vi "Init Messaging.vi"(8 "error in (no error)":errorcluster, 11 "LV Server in":refnum<class "LV Server.lvclass">) -> (0 "error out":errorcluster, 3 "LV Server out":refnum<class "LV Server.lvclass">)   [LabVIEW 2020, in "LV Server.lvclass"]
uses:
  LV Server.lvclass
  <vilib>/IlluminatedG/IG WebSocket Stream/Stream-Websocket/Websocket Server/Websocket Server.lvclass
  C:/Program Files (x86)/National Instruments/LabVIEW 2020/vi.lib/IlluminatedG/lv-stream/Endpoint/Endpoint.lvclass
  <vilib>/IlluminatedG/lv-stream-tcp/TCP Server/TCP Server.lvclass
  Common/Message ID.ctl
  <vilib>/IlluminatedG/lv-msg-simple/Stream-Simple-Msg/Format.ctl
  LV Server.lvclass/LV Server.ctl
  a2551aa6-fa0e-45db-bb02-4b480539a16d.vi
  Connection State Callback.vi
  Message Callback.vi
  <vilib>/IlluminatedG/lv-stream/Endpoint/Endpoint.lvclass
  <vilib>/IlluminatedG/lv-msg-simple/Stream-Simple-Msg/Manager/Manager.lvclass
  <vilib>/IlluminatedG/lv-stream-tcp/Stream-TCP.lvlib
  Common/Common.lvlib
  <vilib>/IlluminatedG/lv-msg-simple/Stream-Simple-Msg/Stream-Simple-Msg.lvlib
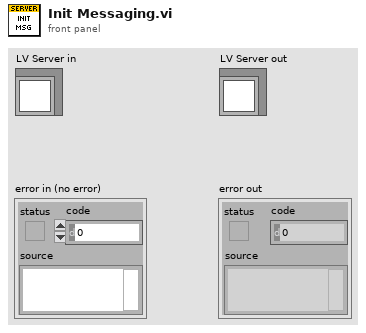
[diagram p1: front panel]
types:
  T1 = typedef "Stream-Simple-Msg.lvlib/Format.ctl" = enum16{"LabVIEW Binary", "JSON"}
  T2 = typedef "Common.lvlib/Message ID.ctl" = enum16{"Timer State", "Timer Value", "Timer Start", "Timer Pause", "Timer Reset", "Timer Init"}
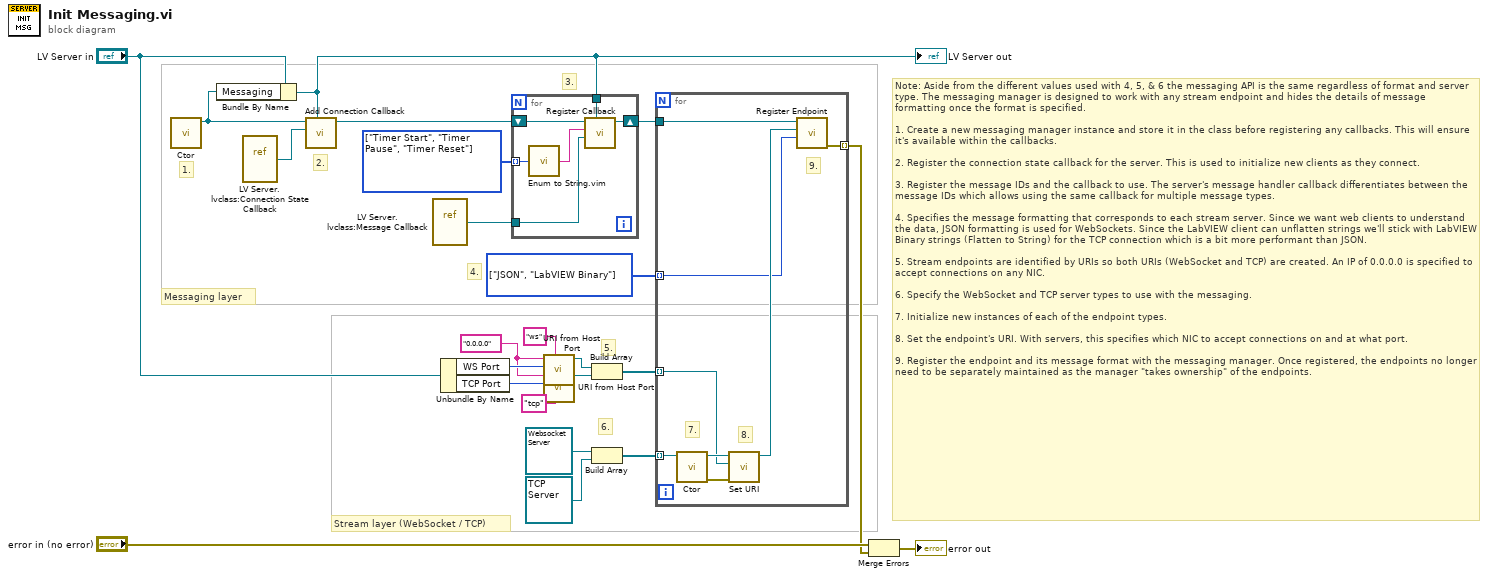
[diagram p0: block diagram]
diagram:
  w4 = T1[] [enum."JSON", enum."LabVIEW Binary"] items=["LabVIEW Binary", "JSON"] ("Format (LabVIEW Binary)")
  w6 = T2[] [enum."Timer Start", enum."Timer Pause", enum."Timer Reset"] items=["Timer State", "Timer Value", "Timer Start", "Timer Pause", "Timer Reset", "Timer Init"]
  w18 = "0.0.0.0"
  # "Stream layer (WebSocket / TCP)"
  # "Messaging layer"
  # "Note: Aside from the different values used with 4, 5, & 6 the messaging API is the same regardless of format and server type. The messaging manager is designed to work with any stream endpoint and hides the details of message formatting once the format is specified.\n\n1. Create a new messaging manager instance and store it in the class before registering any callbacks. This will ensure it's available within the callbacks.\n\n2. Register the connection state callback for the server. This is used to initialize new clients as they connect.\n\n3. Register the message IDs and the callback to use. The server's message handler callback differentiates between the message IDs which allows using the same callback for multiple message types.\n\n4. Specifies the message formatting that corresponds to each stream server. Since we want web clients to understand the data, JSON formatting is used for WebSockets. Since the LabVIEW client can unflatten strings we'll stick with LabVIEW Binary strings (Flatten to String) for the TCP connection which is a bit more performant than JSON.\n\n5. Stream endpoints are identified by URIs so both URIs (WebSocket and TCP) are created. An IP of 0.0.0.0 is specified to accept connections on any NIC.\n\n6. Specify the WebSocket and TCP server types to use with the messaging.\n\n7. Initialize new instances of each of the endpoint types.\n\n8. Set the endpoint's URI. With servers, this specifies which NIC to accept connections on and at what port.\n\n9. Register the endpoint and its message format with the messaging manager. Once registered, the endpoints no longer need to be separately maintained as the manager \"takes ownership\" of the endpoints."
  # "6."
  # "5."
  # "4."
  # "3."
  # "2."
  # "1."
  n1 = call <vilib>:"Ctor.vi"() -> ("Manager out"=w10:refnum<class "Manager.lvclass">)  [unwired: 10 in, 1 out]
  n2 = Bundle By Name(cluster="LV Server in", "Messaging"=w10) -> (w1:refnum<class "LV Server.lvclass">)
  "LV Server out" <- w1
  n3 = vi-ref "LV Server.lvclass:Connection State Callback.vi"() -> (w9:refnum<vi>)
  n4 = call <vilib>:"Add Connection Callback.vi"("Owner"=w1, "Callback"=w9, "Manager in"=w10) -> ("Manager out"=w8:refnum<class "Manager.lvclass">)  [unwired: 7 in, 1 out]
  n5 = vi-ref "LV Server.lvclass:Message Callback.vi"() -> (w7:refnum<vi>)
  n6 = Unbundle By Name("LV Server in") -> ("WS Port"=w21:u16, "TCP Port"=w19:u16)
  n7 = for {
    tunnel: w7 -> [w28]
    shift-right: [w27] -> w5
    shift-left: w8 -> [w29]
    tunnel: w6 -> [w25] mode=indexing
    tunnel: w1 -> [w24]
    n8 = call "Enum to String.vim"("Enum"=w25) -> ("Enum String"=w26:string)
    n9 = call <vilib>:"Register Callback.vi"("Owner"=w24, "Callback"=w28, "Message ID"=w26, "Manager in"=w29) -> ("Manager out"=w27:refnum<class "Manager.lvclass">)  [unwired: 6 in, 1 out]
  }
  n10 = call <vilib>:"URI from Host Port.vi"("Scheme (tcp)"="ws", "Port"=w21, "Host"=w18) -> ("URI"=w16:refnum<class "URI.lvclass">)  [unwired: 8 in]
  n11 = call <vilib>:"URI from Host Port.vi"("Scheme (tcp)"="tcp", "Port"=w19, "Host"=w18) -> ("URI"=w15:refnum<class "URI.lvclass">)  [unwired: 8 in]
  n12 = Build Array(w16, w15) -> (w13:refnum<class "URI.lvclass">[])
  n13 = Build Array(refnum<class "Websocket Server.lvclass"> refnum ("Websocket Server in"), refnum<class "TCP Server.lvclass"> refnum ("TCP Server in")) -> (w14:refnum<class "Endpoint.lvclass">[])
  n14 = for {
    tunnel: w13 -> [w35] mode=indexing
    tunnel: w14 -> [w37] mode=indexing
    tunnel: w4 -> [w31] mode=indexing
    tunnel: w5 -> [w33]
    tunnel: [w30] -> w2 mode=indexing
    # "9."
    # "8."
    # "7."
    n15 = call-dynamic <vilib>:"Ctor.vi"("Endpoint in"=w37) -> ("error out"=w34:errorcluster, "Endpoint out"=w36:refnum<class "Endpoint.lvclass">)  [unwired: 9 in]
    n16 = call <vilib>:"Set URI.vi"("error in (no error)"=w34, "URI"=w35, "Endpoint in"=w36) -> ("Endpoint out"=w32:refnum<class "Endpoint.lvclass">)  [unwired: 7 in, 1 out]
    n17 = call <vilib>:"Register Endpoint.vi"("Format (LabVIEW Binary)"=w31, "Stream:Endpoint"=w32, "Manager in"=w33) -> ("error out"=w30:errorcluster)  [unwired: 7 in, 1 out]
  }
  n18 = Merge Errors("error in (no error)", w2) -> (→"error out":errorcluster)
